vi "Get Shape Position.vi"(8 "error in (no error)":errorcluster, 11 "Shape refnum":refnum<k7>) -> (0 "error out":errorcluster, 3 "Shapre refnum out":refnum<k7>)   [LabVIEW 2020, in "lvpptx.lvlib"]
uses:
  lvpptx.lvlib
  Position.ctl
panel:
  out "Position":T1
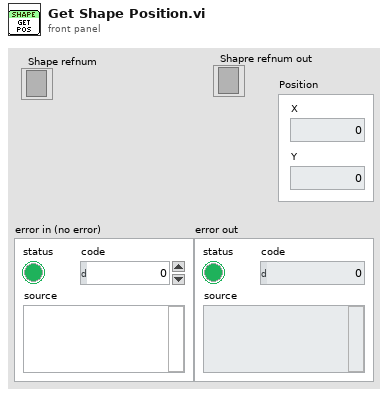
[diagram p1: front panel]
types:
  T1 = typedef "lvpptx.lvlib/Position.ctl" = cluster{"X":dbl, "Y":dbl}
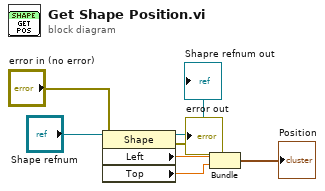
[diagram p0: block diagram]
diagram:
  n1 = property class="Shape"(reference="Shape refnum", error in="error in (no error)") -> (reference out=→"Shapre refnum out":refnum<k7>, error out=→"error out":errorcluster, "Left"=w6:sgl, "Top"=w5:sgl)
  n2 = Bundle("Left"=w6, "Top"=w5) -> (→"Position":cluster{"Left":sgl, "Top":sgl})  [unwired: 1 in]
